vi "CSM - Send Message and Wait for Reply(SimMode).vi"(6 "Response Timeout(5000ms)":i32=5000, 8 "Error In (no error)":errorcluster, 9 "Target Module":string="A", 10 "Arguments (\"\")":string, 11 "State":string="DoA") -> (0 "error out":errorcluster, 2 "Response":string="DoA")   [LabVIEW 2017, in "Communicable State Machine.lvlib"]
doc: "Send a message to CSM specified and wait for the reply with timeout.\n\n<b>Inputs:</b>\n - <b>Target Module</b>: Target CSM Module name.\n - <b>State</b>: Message to send\n - <b>Arguments (\"\")</b>: Argument of the message.\n - <b>Response Timeout(5000ms)</b>: Timeout for waiting the response.\n - <b>Error In (no error)</b>: Error cluster\n\n<b>Outputs:</b>\n - <b>Arguments</b>: Response returned.\n - <b>error out</b>: Error cluster"
uses:
  Communicable State Machine.lvlib
  CSM - Message Type.ctl
  _Support/Priority Queue/Priority Queue.lvclass/Priority Queue.ctl
  _Support/Process/CSMP-Async Call.vi
  _Support/GlobalEvent/GEvt-Generate Status Log.vi
  _Support/Process/CSMP-Broadcast.vi
  _Support/GlobalEvent/GEvt-Generate Interrupt Log.vi
  _Support/GlobalEvent/GEvt-Generate Register Log.vi
  _Support/Process/CSMP-Register Status.vi
  _Support/GlobalEvent/GEvt-Generate Unregister Log.vi
  _Support/Process/CSMP-Unregister Status.vi
  _Support/Process/CSMP-Sync Call.vi
  _Support/CSMQ/_CSMObj-Unlock.vi
  _Support/Process/CSMP-PostPostMsg.vi
  _Support/Process/CSMP-PostSendMsg.vi
  _Support/CSMQ/_CSMObj-Lock State.vi
  _Support/Common/Splite Reason String Part.vi
  _Support/Common/Trim Single line Text.vi
  CSM - Convert Argument to Error.vi
  _Support/CSMQ/_CSMOFGV Release.vi
  _Support/Common/Remove Comments from Line.vi
  _Support/Common/Splite Single-line Message.vi
  _Support/Common/Parse Next Single-line State.vi
  _Support/CSMQ/_CSMOFGV Dequeue.vi
  CSM - Convert Error to Argument.vi
  _Support/CSMQ/_CSMObj-Log Error if in a Remote Session.vi
  _Support/GlobalEvent/GEvt-Generate State Change Log.vi
  _Support/GlobalEvent/GEvt-Generate Remaining States Log.vi
  _Support/GlobalEvent/GEvt-Generate Module Destroyed Log.vi
  _Support/GlobalEvent/GEvt-Generate Complete Log.vi
  _Support/GlobalEvent/GEvt-Generate Module Created Log.vi
  _Support/CSMQ/_CSMObj-Message Check.vi
  _Support/CSMQ/_CSMObj-Enqueue Cross-Module Message.vi
  _Support/CSMQ/_CSMOFGV Get.vi
  _Support/FGV-BroadcastRegistry/Cache-Broadcast Registry Search Result.vi
  CSM - Register Status Change.vi
  CSM - Unregister Status Change.vi
  _Support/Common/Hex Str to U8 Data.vi
  CSM - Revert Arguments-Safe String.vi
  <vilib>/addons/_JKI Toolkits/State Machine/_JKI_lib_State_Machine.llb/Add State(s) to Queue__JKI_lib_State_Machine.vi
  Utility/Build Internal State String.vi
  _Support/Common/Concatenate State with Arguments.vi
  _Support/Common/U8 Data to Hex Str.vi
  _Support/Priority Queue/Dequeue Element.vi
  CSM - Make String Arguments Safe.vi
  _Support/Priority Queue/Enqueue Element.vi
  CSM - Keywords.vi
  _Support/CSMQ/_CSMOFGV.vi
  _Support/Error/CSM Not Allowed Message.vi
  _Support/FGV-BroadcastRegistry/FGV-BroadcastRegistry.vi
  _Support/Message/Parse Unregister Message.vi
  _Support/Message/Parse Register Message.vi
  _Support/BroadcastRegistry/HelperVI/Broadcast Item Key.vi
  _Support/FGV-BroadcastRegistry/global-Broadcast Cache Change Flag.vi
  _Support/FGV-BroadcastRegistry/global-CSMQ FGV Change Flag.vi
  _Support/GlobalEvent/FGV-StatusChangeEventRef.vi
  _Support/CSMQ/_CSMOFGV Obtain.vi
  _Support/GlobalEvent/FGV-GlobalEventRef.vi
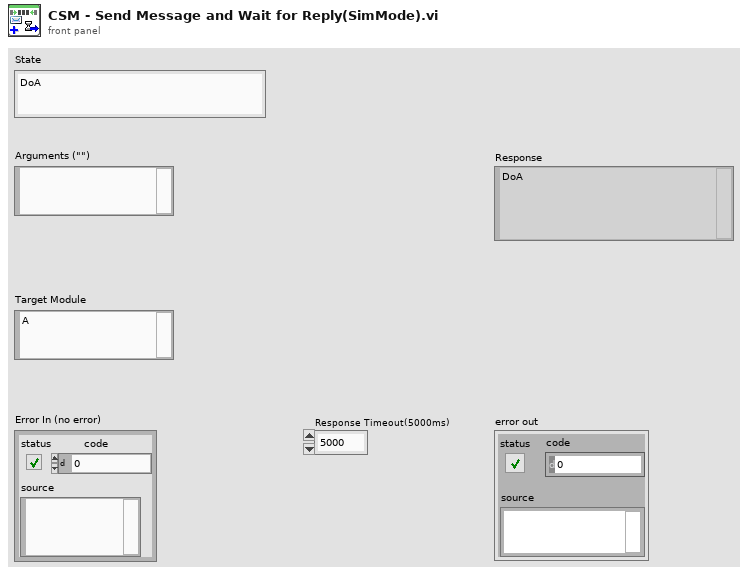
[diagram p1: front panel]
types:
  T1 = typedef "Communicable State Machine.lvlib/CSM - Message Type.ctl" = enum16{"Async", "Async without Reply", "Sync"}
  T2 = typedef "Communicable State Machine.lvlib/_CSM_Response Source Message.ctl" = cluster{"‘State":string, "’Arguments":string, "’Error":errorcluster}
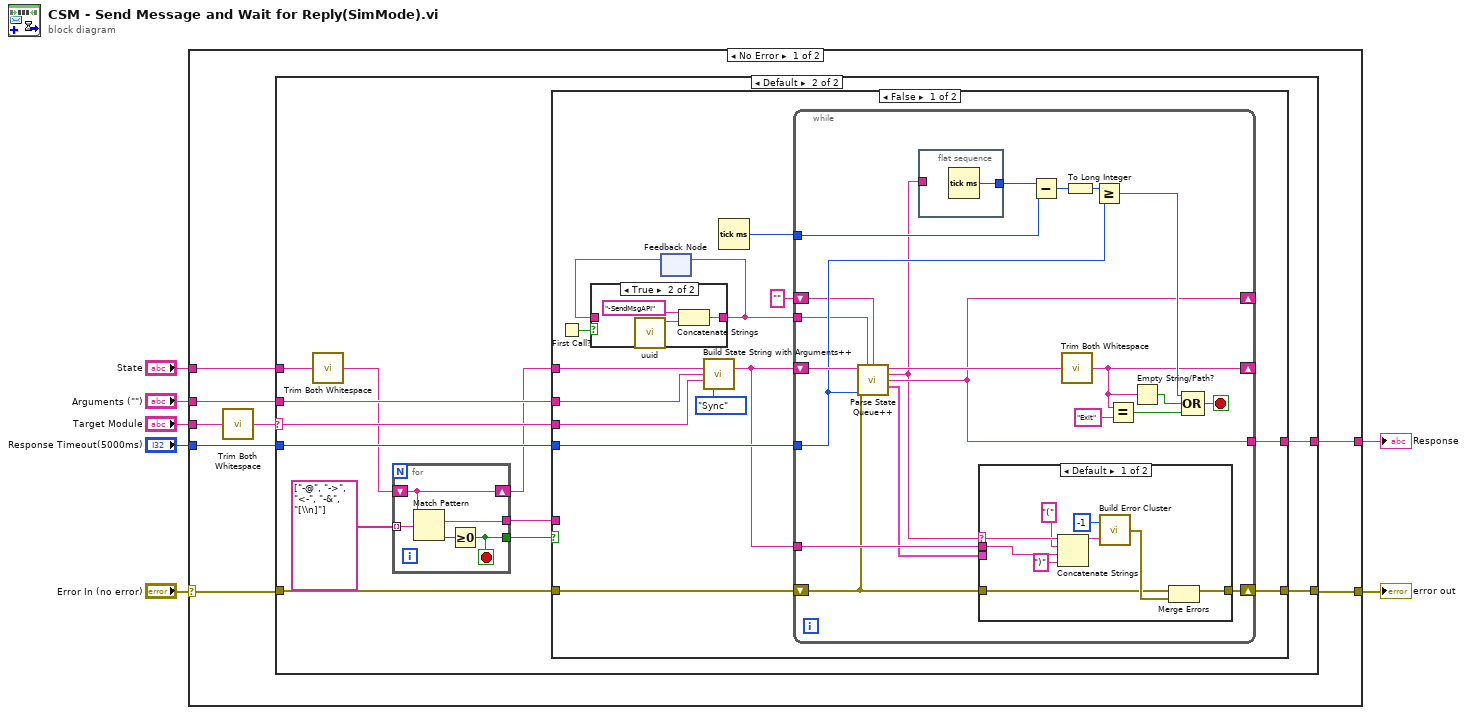
[diagram p0: block diagram]
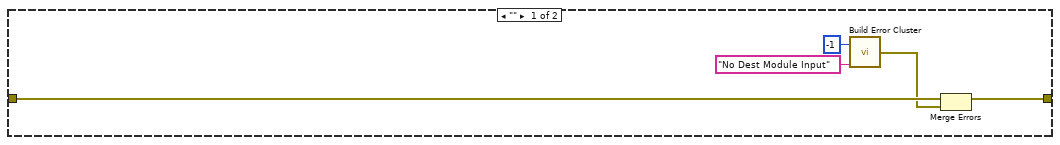
[diagram p2: hidden frame]
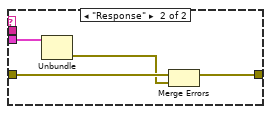
[diagram p4: hidden frame]
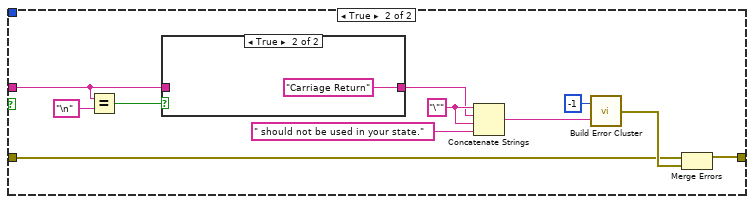
[diagram p5: hidden frame]
diagram:
  n1 = case shown="No Error" "Error In (no error)" {
    selector: "Error In (no error)" -> [w14 w104]
    tunnel: "State" -> [w15 _]
    tunnel: "Response Timeout(5000ms)" -> [w13 _]
    tunnel: [w9 w104] -> w4
    tunnel: [w12 _] -> w3
    tunnel: "Target Module" -> [w11 _]
    tunnel: "Arguments (\"\")" -> [w10 _]
    frame No Error {
      n2 = call "Trim Both Whitespace.vi"("string"=w11) -> ("trimmed string"=w8:string)  [unwired: 1 in]
      n3 = case shown="Default" w8 {
        selector: w8 -> [_ w29]
        tunnel: w14 -> [w18 w32]
        tunnel: w13 -> [_ w31]
        tunnel: [_ w30] -> w12
        tunnel: w10 -> [_ w28]
        tunnel: [w17 w27] -> w9
        tunnel: w15 -> [_ w26]
        frame "" {
          n4 = call "Build Error Cluster.vi"("String to Prepend to source (\"\")"="No Dest Module Input" ("String to Prepend to source (\"\")"), "code"=-1) -> ("error out"=w16:errorcluster)
          n5 = Merge Errors(w18, w16) -> (w17:errorcluster)
        }
        frame Default {
          n6 = call "Trim Both Whitespace.vi"("string"=w26) -> ("trimmed string"=w21:string)  [unwired: 1 in]
          n7 = for {
            shift-right: [w103] -> w25
            shift-left: w21 -> [w103]
            tunnel: string[] ["-@", "->", "<-", "-&", "[\\n]"] -> [w102] mode=indexing
            tunnel: [w100] -> w23
            tunnel: [w99] -> w24
            stop <- w99 stop-if-true
            n8 = Match Pattern(string=w103, regular expression=w102) -> (match substring=w100:string, offset past match=w101:i32)  [unwired: 1 in, 2 out]
            n9 = Greater Or Equal To 0?(x=w101) -> (x >= 0?=w99:bool)
          }
          n10 = case shown="False" w24 {
            tunnel: w32 -> [w46 w92]
            tunnel: w31 -> [w45 _]
            tunnel: [w43 _] -> w30
            tunnel: w29 -> [w42 _]
            tunnel: w28 -> [w41 _]
            tunnel: [w40 w93] -> w27
            tunnel: w25 -> [w35 _]
            tunnel: w23 -> [_ w88]
            frame False {
              n11 = First Call?() -> (First Call?: T/F=w37:bool)
              n12 = feedback #1() -> (w36:string)  [unwired: 1 in]
              n13 = case shown="True" w37 {
                tunnel: [w47 w48] -> w38
                tunnel: w36 -> [w47 _]
                frame False {
                }
                frame True {
                  n14 = call "uuid.vi"() -> ("UUID"=w49:string)  [unwired: 11 in]
                  n15 = Concatenate Strings("-SendMsgAPI" ("Name(\"\" to use uuid)"), w49) -> (w48:string)
                }
              }
              n16 = feedback-in #1(w38) -> ()
              n17 = call "Build State String with Arguments++.vi"("State"=w35, "Arguments (\"\")"=w41, "Target Module (\"\")"=w42, "Type"=CSM_-_Message_Type."Sync") -> ("State with Arguments"=w39:string)  [unwired: 11 in]
              n18 = Tick Count (ms)() -> (millisecond timer value=w44:u32)
              n19 = while {
                shift-right: [w52] -> _
                shift-left: w39 -> [w71]
                tunnel: w45 -> [w65]
                tunnel: w44 -> [w68]
                tunnel: [w62] -> w43
                shift-right: [w62] -> _
                shift-left: "" ("Arguments") -> [w61]
                tunnel: w38 -> [w60]
                tunnel: w39 -> [w58]
                shift-right: [w57] -> w40
                shift-left: w46 -> [w56]
                stop <- w67 stop-if-true
                n20 = call "Parse State Queue++.vi"("State Queue"=w71, "Name(\"\" to use uuid)"=w60, "Response Arguments"=w61, "Error In (no error)"=w56, "Response Timeout(5000ms)"=w65) -> ("Remaining States"=w70:string, "Current State"=w59:string, "Arguments"=w62:string, ">> Response Source Message >>"=w51:T2)  [unwired: 5 in, 2 out]
                n21 = flat-sequence {
                  tunnel: [w85] -> w69
                  tunnel: w59 -> [_]
                  frame #0 {
                    n22 = Tick Count (ms)() -> (millisecond timer value=w85:u32)
                  }
                }
                n23 = case shown="Default" w59 {
                  selector: w59 -> [w79 _]
                  tunnel: [w76 w82] -> w57
                  tunnel: w56 -> [w75 w84]
                  tunnel: w58 -> [w74 _]
                  tunnel: w51 -> [_ w83]
                  frame Default {
                    n24 = Concatenate Strings(w79, "(" ("string"), w74, ")" ("string")) -> (w78:string)
                    n25 = call "Build Error Cluster.vi"("String to Prepend to source (\"\")"=w78, "code"=-1) -> ("error out"=w77:errorcluster)
                    n26 = Merge Errors(w75, w77) -> (w76:errorcluster)
                  }
                  frame "Response" {
                    n27 = Unbundle(w83) -> ("’Error"=w81:errorcluster)  [unwired: 2 out]
                    n28 = Merge Errors(w84, w81) -> (w82:errorcluster)
                  }
                }
                n29 = Subtract(x=w69, y=w68) -> (x-y=w66:u32)
                n30 = call "Trim Both Whitespace.vi"("string"=w70) -> ("trimmed string"=w52:string)  [unwired: 1 in]
                n31 = To Long Integer(number=w66) -> (32bit integer=w63:i32)
                n32 = Greater Or Equal?(x=w63, y=w65) -> (x >= y?=w64:bool)
                n33 = Equal?(x=w52, y="Exit" ("State(s) at Back (\"\")")) -> (x = y?=w55:bool)
                n34 = Empty String/Path?(string/path=w52) -> (empty?=w53:bool)
                n35 = Compound Arithmetic op=OR(w64, w53, w55) -> (w67:bool)
              }
            }
            frame True {
              w90 = "\"" ("string")
              n36 = Equal?(x=w88, y="\n" ("regular expression")) -> (x = y?=w86:bool)
              n37 = case shown="True" w86 {
                tunnel: [w97 "Carriage Return" ("State")] -> w89
                tunnel: w88 -> [w97 _]
                frame False {
                }
                frame True {
                }
              }
              n38 = Concatenate Strings(w90, w89, w90, " should not be used in your state." ("String to Prepend to source (\"\")")) -> (w91:string)
              n39 = call "Build Error Cluster.vi"("String to Prepend to source (\"\")"=w91, "code"=-1) -> ("error out"=w94:errorcluster)
              n40 = Merge Errors(w92, w94) -> (w93:errorcluster)
            }
          }
        }
      }
    }
    frame Error {
    }
  }
  "error out" <- w4
  "Response" <- w3
